vi "DriveForTime.vi"() -> ()   [LabVIEW 2018]
uses:
  Framework/Robot Global Data.vi
panel:
  in  "NoWait":bool
  in  "Time":dbl
  in  "Speed":dbl
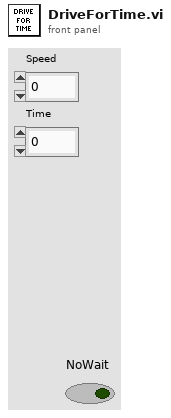
[diagram p1: front panel]
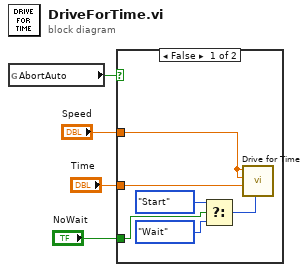
[diagram p0: block diagram]
diagram:
  n1 = global read "Robot Global Data.vi" "AbortAuto"() -> (w1:bool)
  n2 = case shown="False" w1 {
    tunnel: "Speed" -> [w7 _]
    tunnel: "Time" -> [w6 _]
    tunnel: "NoWait" -> [w5 _]
    frame False {
      n3 = Select(t=enum16{"Start", "Wait"}."Start", s=w5, f=enum16{"Start", "Wait"}."Wait" ("Synchronication")) -> (s? t:f=w10:enum16{"Start", "Wait"})
      n4 = call "Drive for Time.vi"("Synchronization"=w10, "Seconds"=w6, "Right Speed"=w7, "Left Speed"=w7) -> ()  [unwired: 6 in, 2 out]
    }
    frame True {
    }
  }
